vi "Request Data JSON.vi"(8 "error in (no error)":errorcluster, 11 "SetPersistentData in":refnum<class "SetPersistentData.lvclass">) -> (0 "error out":errorcluster, 2 "Request Data JSON":string, 3 "SetPersistentData out":refnum<class "SetPersistentData.lvclass">)   [LabVIEW 2020, in "obs-websocket.lvlib" / "SetPersistentData.lvclass"]
uses:
  SetPersistentData.lvclass
  SetPersistentData.lvclass/SetPersistentData.ctl
  c20c4316-0aeb-4c48-95ef-8f1ae9b8bf61.vi
  <vilib>/JDP Science/JSONtext/Variant to JSON Text.vi
  <vilib>/JDP Science/JSONtext/LVClass Serializer/JSONtext LVClass Serializer.lvclass
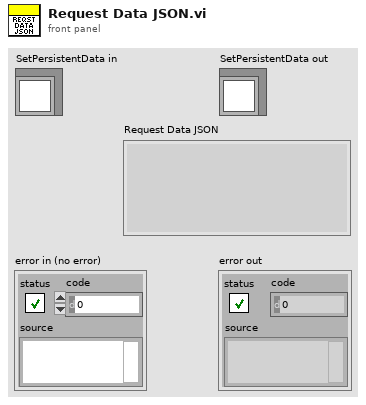
[diagram p1: front panel]
types:
  T1 = cluster{"realm":string, "slotName":string, "slotValue":string}
  T2 = typedef "obs-websocket.lvlib/Data Realm.ctl" = enum16{"Global", "Profile"}
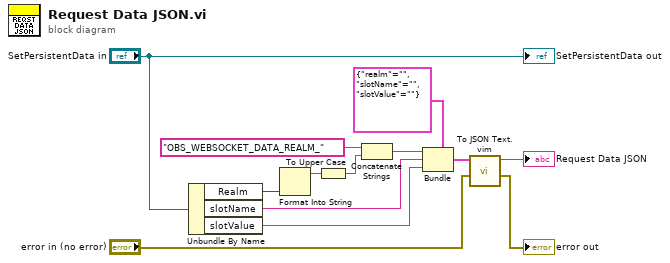
[diagram p0: block diagram]
diagram:
  n1 = Unbundle By Name("SetPersistentData in") -> ("Realm"=w13:T2, "slotName"=w6:string, "slotValue"=w5:string)
  n2 = Format Into String(w13) -> (resulting string=w12:string)  [unwired: 3 in, 1 out]
  n3 = To Upper Case(1:w12) -> (0:w11:string)
  n4 = Concatenate Strings("OBS_WEBSOCKET_DATA_REALM_" ("string"), w11) -> (w7:string)
  n5 = Bundle(cluster=T1 {"realm"="", "slotName"="", "slotValue"=""}, "realm"=w7, "slotName"=w6, "slotValue"=w5) -> (w4:T1)
  n6 = call "To JSON Text.vim"("error in (no error)"="error in (no error)", "Anything"=w4) -> ("error out"=→"error out":errorcluster, "<JSON>"=→"Request Data JSON":string)  [unwired: 8 in]
  "SetPersistentData out" <- "SetPersistentData in"
